vi "Creators Created Events.vi"(8 "Created Event Alias":string, 9 "Priority?":bool, 10 "Msg Strategy":refnum<class "Msg Strategy.lvclass">, 11 "Template Event in":refnum<class "Template Event.lvclass">) -> (3 "Template Event out":refnum<class "Template Event.lvclass">)   [LabVIEW 2021, in "_Template.lvlib" / "Templates.lvlib" / "Template Event.lvlib" / "Template Event.lvclass"]
uses:
  <vilib>/jettl/jettl/jettl/Msg Strategy/Msg Strategy.lvclass
  Template Event.lvclass
  Template Event.lvclass/Template Event.ctl
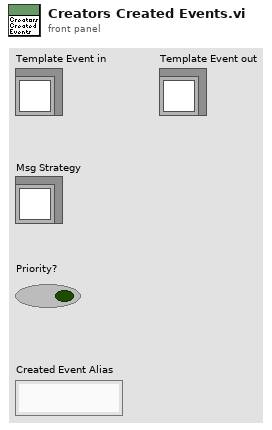
[diagram p1: front panel]
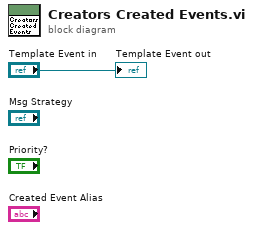
[diagram p0: block diagram]
diagram:
  "Template Event out" <- "Template Event in"
